vi "UI Controls.vi"(0 "Auto Refs":refnum<vi>[](array[refnum]), 1 "Setup":bool, 5 "Manual Refs":refnum<vi>[](array[refnum]), 7 "Script Refs":refnum<vi>[](array[refnum]), 9 "Page Refs In":refnum<vi>, 12 "Auto/Man/Script Refs":refnum<vi>) -> (4 "Auto Refs":refnum<vi>[](array[refnum]), 6 "Manual Refs":refnum<vi>[](array[refnum]), 8 "Script Refs":refnum<vi>[](array[refnum]), 10 "Page Refs Out":refnum<vi>, 14 "Auto/Man/Script Refs":refnum<vi>)   [LabVIEW 2023]
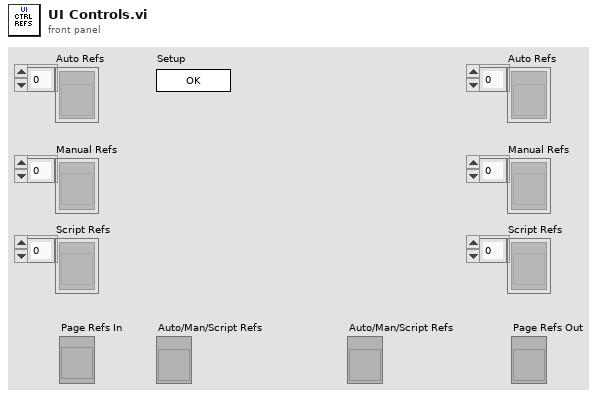
[diagram p1: front panel]
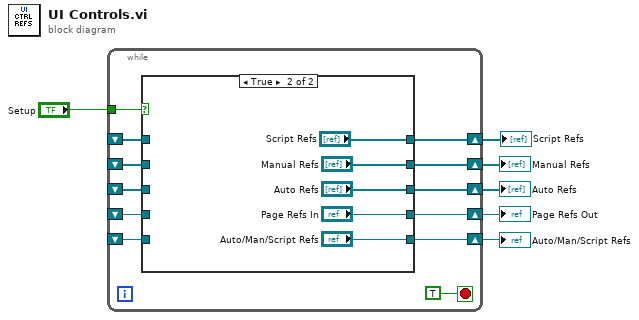
[diagram p0: block diagram]
diagram:
  n1 = while {
    tunnel: "Setup" -> [w18]
    shift-right: [w16] -> w5
    shift-left: _ -> [w14]
    shift-right: [w15] -> w4
    shift-left: _ -> [w13]
    shift-right: [w12] -> w2
    shift-left: _ -> [w10]
    shift-right: [w11] -> w3
    shift-left: _ -> [w9]
    shift-right: [w8] -> w1
    shift-left: _ -> [w7]
    stop <- TRUE stop-if-true
    n2 = case shown="True" w18 {
      tunnel: [w23 "Manual Refs"] -> w16
      tunnel: [w22 "Auto Refs"] -> w15
      tunnel: w14 -> [w23 _]
      tunnel: w13 -> [w22 _]
      tunnel: [w21 "Page Refs In"] -> w12
      tunnel: [w20 "Auto/Man/Script Refs"] -> w11
      tunnel: w10 -> [w21 _]
      tunnel: w9 -> [w20 _]
      tunnel: [w19 "Script Refs"] -> w8
      tunnel: w7 -> [w19 _]
      frame False {
      }
      frame True {
      }
    }
  }
  "Manual Refs" <- w5
  "Auto Refs" <- w4
  "Auto/Man/Script Refs" <- w3
  "Page Refs Out" <- w2
  "Script Refs" <- w1
